vi "Format Inv Data.vi"(11 "logData":T1) -> (2 "No Time Info":string[](array[string]), 3 "Time Info Included":string[](array[string]))   [LabVIEW 2014]
uses:
  Washer HCC/Washer HCC NEWFI/Type Definitions/HCC_logData.ctl
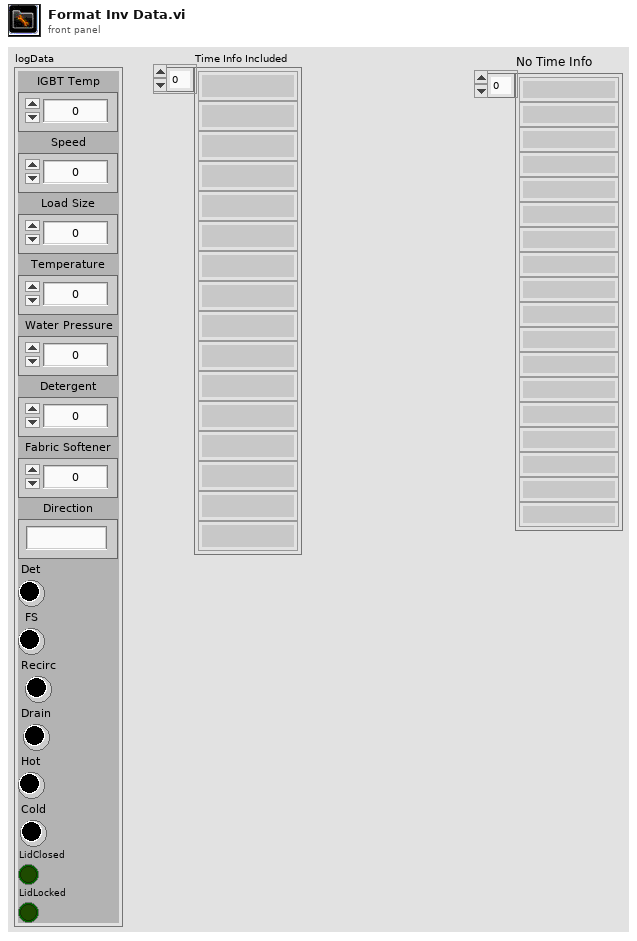
[diagram p1: front panel]
types:
  T1 = typedef "HCC_logData.ctl" = cluster{"IGBT Temp":u8, "Speed":u32, "Load Size":u32, "Temperature":u8, "Water Pressure":u32, "Detergent":u32, "Fabric Softener":u32, "Direction":string, "Det":bool, "FS":bool, "Recirc":bool, "Drain":bool, "Hot":bool, "Cold":bool, "LidClosed":bool, "LidLocked":bool}
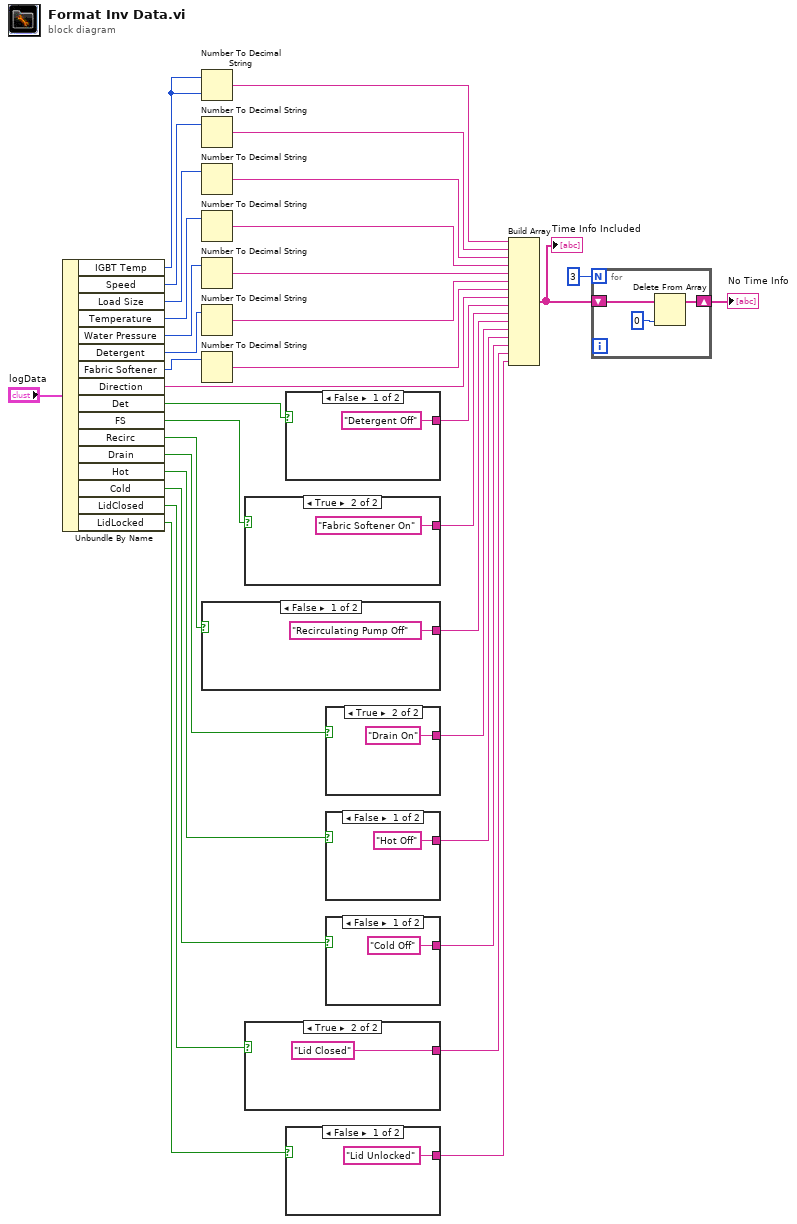
[diagram p0: block diagram]
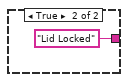
[diagram p2: hidden frame]
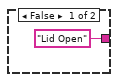
[diagram p3: hidden frame]
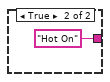
[diagram p4: hidden frame]
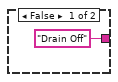
[diagram p5: hidden frame]
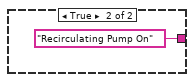
[diagram p6: hidden frame]
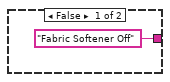
[diagram p7: hidden frame]
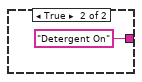
[diagram p8: hidden frame]
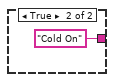
[diagram p9: hidden frame]
diagram:
  n1 = Unbundle By Name("logData") -> ("IGBT Temp"=w34:u8, "Speed"=w32:u32, "Load Size"=w31:u32, "Temperature"=w30:u8, "Water Pressure"=w29:u32, "Detergent"=w35:u32, "Fabric Softener"=w28:u32, "Direction"=w12:string, "Det"=w27:bool, "FS"=w26:bool, "Recirc"=w25:bool, "Drain"=w24:bool, "Hot"=w23:bool, "Cold"=w22:bool, "LidClosed"=w21:bool, "LidLocked"=w20:bool)
  n2 = Number To Decimal String(number=w34, width (-)=w34) -> (decimal integer string=w19:string)
  n3 = Number To Decimal String(number=w32) -> (decimal integer string=w18:string)  [unwired: 1 in]
  n4 = Number To Decimal String(number=w31) -> (decimal integer string=w17:string)  [unwired: 1 in]
  n5 = Number To Decimal String(number=w30) -> (decimal integer string=w16:string)  [unwired: 1 in]
  n6 = Number To Decimal String(number=w29) -> (decimal integer string=w15:string)  [unwired: 1 in]
  n7 = Number To Decimal String(number=w35) -> (decimal integer string=w14:string)  [unwired: 1 in]
  n8 = Number To Decimal String(number=w28) -> (decimal integer string=w13:string)  [unwired: 1 in]
  n9 = case shown="False" w25 {
    tunnel: ["Recirculating Pump Off" "Recirculating Pump On"] -> w9
    frame False {
    }
    frame True {
    }
  }
  n10 = case shown="True" w26 {
    tunnel: ["Fabric Softener Off" "Fabric Softener On"] -> w10
    frame False {
    }
    frame True {
    }
  }
  n11 = case shown="True" w21 {
    tunnel: ["Lid Open" "Lid Closed"] -> w5
    frame False {
    }
    frame True {
    }
  }
  n12 = case shown="False" w27 {
    tunnel: ["Detergent Off" "Detergent On"] -> w11
    frame False {
    }
    frame True {
    }
  }
  n13 = case shown="False" w20 {
    tunnel: ["Lid Unlocked" "Lid Locked"] -> w4
    frame False {
    }
    frame True {
    }
  }
  n14 = case shown="True" w24 {
    tunnel: ["Drain Off" "Drain On"] -> w8
    frame False {
    }
    frame True {
    }
  }
  n15 = case shown="False" w23 {
    tunnel: ["Hot Off" "Hot On"] -> w7
    frame False {
    }
    frame True {
    }
  }
  n16 = case shown="False" w22 {
    tunnel: ["Cold Off" "Cold On"] -> w6
    frame False {
    }
    frame True {
    }
  }
  n17 = Build Array(w19, w18, w17, w16, w15, w14, w13, w12, w11, w10, w9, w8, w7, w6, w5, w4) -> (w3:string[])
  "Time Info Included" <- w3
  n18 = for {
    N: 3 -> [_]
    shift-right: [w52] -> w1
    shift-left: w3 -> [w54]
    n19 = Delete From Array(array=w54, index=0) -> (array with subset deleted=w52:string[])  [unwired: 1 in, 1 out]
  }
  "No Time Info" <- w1
